vi "Push button.vi"() -> (0 "Air Pressure":bool, 1 "Push Button":T1, 3 "Error":string)   [LabVIEW 2015]
uses:
  Galobal variable_TI.vi
panel:
  in  "Cluster":T1
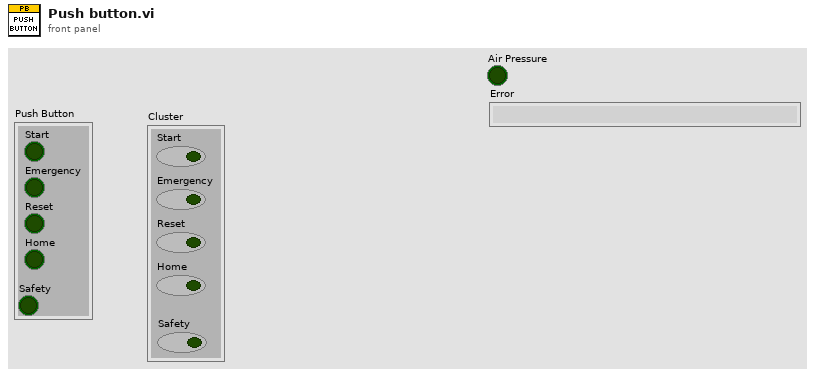
[diagram p1: front panel]
types:
  T1 = cluster{"Start":bool, "Emergency ":bool, "Reset":bool, "Home":bool, "Safety":bool}
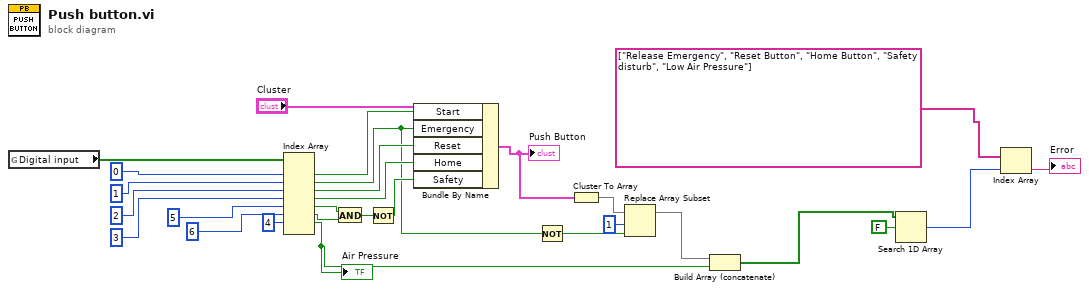
[diagram p0: block diagram]
diagram:
  n1 = global read "Galobal variable_TI.vi" "Digital input"() -> (w24:bool[])
  n2 = Index Array(array=w24, index #1=0 ("index"), index #2=1 ("index"), index #3=2 ("index"), index #4=3 ("index"), index #5=5 ("index"), index #6=6 ("index"), index #7=4 ("index")) -> (element #1=w23:bool, element #2=w7:bool, element #3=w22:bool, element #4=w21:bool, element #5=w18:bool, element #6=w17:bool, element #7=w11:bool)  [unwired: 1 in, 1 out]
  "Air Pressure" <- w11
  n3 = And(x=w18, y=w17) -> (x .and. y?=w16:bool)
  n4 = Not(x=w16) -> (.not. x?=w15:bool)
  n5 = Bundle By Name(cluster="Cluster", "Start"=w23, "Emergency"=w7, "Reset"=w22, "Home"=w21, "Safety"=w15) -> (w12:T1)
  "Push Button" <- w12
  n6 = Not(x=w7) -> (.not. x?=w6:bool)
  n7 = Cluster To Array(cluster=w12) -> (array=w5:bool[])
  n8 = Replace Array Subset(array=w5, new element=w6, index=1) -> (w4:bool[])
  n9 = Build Array (concatenate)(w4, w11) -> (w10:bool[])
  n10 = Search 1D Array(1D array=w10, element=FALSE) -> (index of element=w2:i32)  [unwired: 1 in]
  n11 = Index Array(array=string[] ["Release Emergency", "Reset Button", "Home Button", "Safety disturb", "Low Air Pressure"], index=w2) -> (element=→"Error":string)
